vi "Add Subscription.vi"(8 "error in (no error)":errorcluster, 9 "SessionMailbox":refnum<queue>, 10 "Topic Subscription":T1, 11 "MQTT_Base in":refnum<class "MQTT_Base.lvclass">) -> (0 "error out":errorcluster, 1 "Failed":bool, 3 "MQTT_Base out":refnum<class "MQTT_Base.lvclass">)   [LabVIEW 2013, in "MQTT Server.lvlib" / "MQTT_Base.lvclass"]
uses:
  MQTT_Base.lvclass
  Control Packets/SUBSCRIBE/Topic Subscription -- cluster.ctl
  Control Packets/ControlPacket/QualityOfService -- enum.ctl
  Response -- cluster.ctl
  Control Packets/ControlPacket/ControlPacket.lvclass
  MQTT_Base.lvclass/MQTT_Base.ctl
  Server/Subscription/Subscription.lvclass/Subscription.ctl
  Server/TopicFilter/TopicFilter.lvclass/TopicFilter.ctl
  Server/Subscription/Subscription.lvclass
  Control Packets/SUBSCRIBE/SUBSCRIBE.lvclass
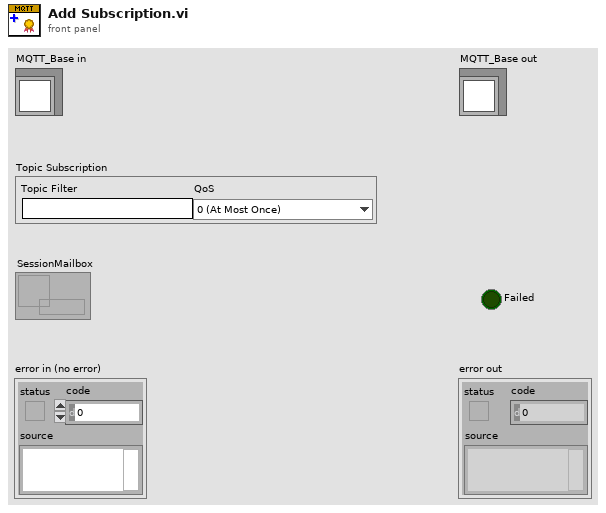
[diagram p1: front panel]
types:
  T1 = typedef "SUBSCRIBE.lvclass/Topic Subscription -- cluster.ctl" = cluster{"Topic Filter":string, "QoS":T2}
  T2 = typedef "ControlPacket.lvclass/QualityOfService -- enum.ctl" = enum16{"0 (At Most Once)", "1 (At Least Once)", "2 (Exactly Once)"}
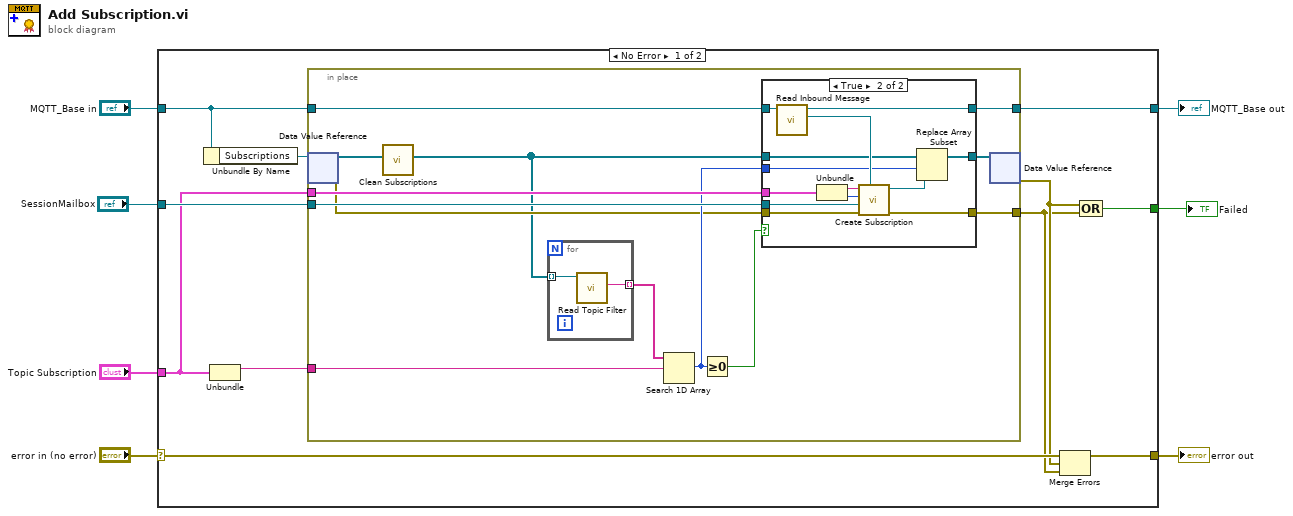
[diagram p0: block diagram]
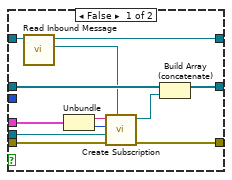
[diagram p2: hidden frame]
diagram:
  n1 = case shown="No Error" "error in (no error)" {
    selector: "error in (no error)" -> [w17 w60]
    tunnel: [w16 w60] -> w6
    tunnel: [w13 w59] -> w4
    tunnel: "MQTT_Base in" -> [w14 w59]
    tunnel: "Topic Subscription" -> [w11 _]
    tunnel: [w8 _] -> w2
    tunnel: "SessionMailbox" -> [w12 _]
    frame No Error {
      n2 = Unbundle By Name(w14) -> ("Subscriptions"=w18:refnum<data-value>)
      n3 = Unbundle(w11) -> ("Topic Filter"=w15:string)  [unwired: 1 out]
      n4 = in-place {
        in-place-border: w15 -> [w28]
        in-place-border: w14 -> [w27]
        in-place-border: [w26] -> w13
        in-place-border: w12 -> [w25]
        in-place-border: w11 -> [w24]
        in-place-border: [w22] -> w9
        n5 = in-place-dvr #1(w18) -> (w20:refnum<class "Subscription.lvclass">[], w21:errorcluster)
        n6 = call "Clean Subscriptions.vi"("Subscriptions in"=w20) -> ("Subscriptions"=w19:refnum<class "Subscription.lvclass">[])  [unwired: 10 in]
        n7 = for {
          tunnel: [w58] -> w30 mode=indexing
          tunnel: w19 -> [w57] mode=indexing
          n8 = call "Read Topic Filter.vi"("Subscription in"=w57) -> ("Topic Filter"=w58:string)  [unwired: 7 in, 3 out]
        }
        n9 = Search 1D Array(1D array=w30, element=w28) -> (index of element=w23:i32)  [unwired: 1 in]
        n10 = Greater Or Equal To 0?(x=w23) -> (x >= 0?=w29:bool)
        n11 = case shown="True" w29 {
          tunnel: [w43 w48] -> w31
          tunnel: w19 -> [w42 w49]
          tunnel: w27 -> [w41 w56]
          tunnel: [w40 w55] -> w26
          tunnel: w25 -> [w37 w53]
          tunnel: w24 -> [w34 w50]
          tunnel: w23 -> [_ w47]
          tunnel: [w33 w46] -> w22
          tunnel: w21 -> [w32 w45]
          frame False {
            n12 = call "Read Inbound Message.vi"("MQTT_Base in"=w41) -> ("Inbound Message"=w38:refnum<user-event>, "MQTT_Base out"=w40:refnum<class "MQTT_Base.lvclass">)  [unwired: 8 in, 1 out]
            n13 = Unbundle(w34) -> ("Topic Filter"=w36:string, "QoS"=w35:T2)
            n14 = call "Create Subscription.vi"("Inbound Message"=w38, "error in (no error)"=w32, "SessionMailbox"=w37, "QoS"=w35, "Topic Filter"=w36) -> ("error out"=w33:errorcluster, "Subscription out"=w39:refnum<class "Subscription.lvclass">)  [unwired: 5 in]
            n15 = Build Array (concatenate)(w42, w39) -> (w43:refnum<class "Subscription.lvclass">[])
          }
          frame True {
            n16 = call "Read Inbound Message.vi"("MQTT_Base in"=w56) -> ("Inbound Message"=w54:refnum<user-event>, "MQTT_Base out"=w55:refnum<class "MQTT_Base.lvclass">)  [unwired: 8 in, 1 out]
            n17 = Unbundle(w50) -> ("Topic Filter"=w52:string, "QoS"=w51:T2)
            n18 = call "Create Subscription.vi"("Inbound Message"=w54, "error in (no error)"=w45, "SessionMailbox"=w53, "QoS"=w51, "Topic Filter"=w52) -> ("error out"=w46:errorcluster, "Subscription out"=w44:refnum<class "Subscription.lvclass">)  [unwired: 5 in]
            n19 = Replace Array Subset(array=w49, new element=w44, index=w47) -> (w48:refnum<class "Subscription.lvclass">[])
          }
        }
        n20 = in-place-dvr #1(w31) -> (w10:errorcluster)  [unwired: 1 out]
      }
      n21 = Merge Errors(w17, w10, w9) -> (w16:errorcluster)
      n22 = Compound Arithmetic op=OR(w10, w9) -> (w8:bool)
    }
    frame Error {
    }
  }
  "error out" <- w6
  "MQTT_Base out" <- w4
  "Failed" <- w2
